vi "Write Global Configuration.vi"(10 "Global Configuration":refnum<data-value>, 11 "EMS Generic in":refnum<class "EMS Generic.lvclass">) -> (3 "EMS Generic out":refnum<class "EMS Generic.lvclass">)   [LabVIEW 2018, in "EMS Generic Actor.lvlib" / "EMS Generic.lvclass"]
uses:
  EMS Generic.lvclass
  EMS Generic.lvclass/EMS Generic.ctl
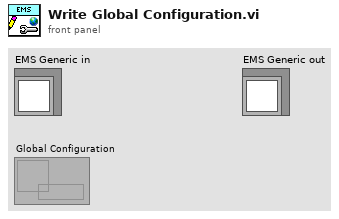
[diagram p1: front panel]
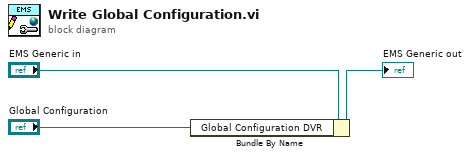
[diagram p0: block diagram]
diagram:
  n1 = Bundle By Name(cluster="EMS Generic in", "Global Configuration DVR"="Global Configuration") -> (→"EMS Generic out":refnum<class "EMS Generic.lvclass">)
